vi "Set Cluster Element Disabled.vi"(6 "Disabled":T1(ring), 8 "error in":errorcluster, 9 "Class To Set":string, 10 "Index":i32, 11 "Cluster":refnum<vi>) -> (0 "error out":errorcluster, 3 "Cluster (dup)":refnum<vi>)   [LabVIEW 2015, in "Utility.lvlib"]
doc: "Used to set the Disabled property of an element of a cluster, referenced via the <b>Index</b> input.\n\nA special mode of operation of this VI is when <b>Index</b> is set to -1. In this case the disabled state is applied to all the controls in the cluster of the specific Class referenced by <b>Class To Set</b>. If this input is empty the class is ignored and the disabled state is applied to all the controls in the cluster. The <b>Class To Set</b> input is not case sensitive."
uses:
  Utility.lvlib
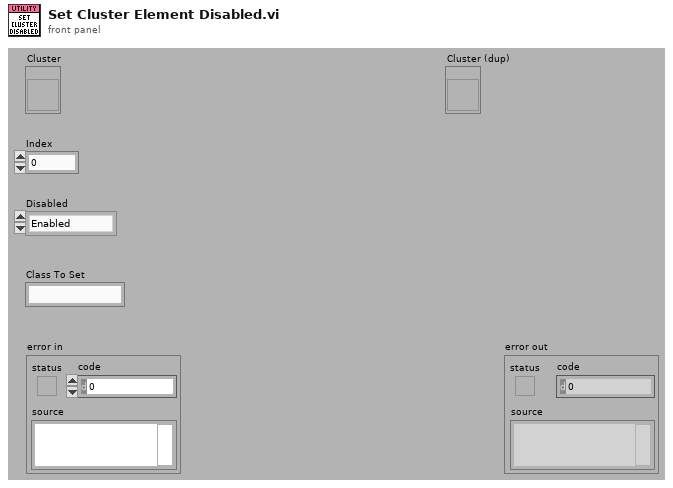
[diagram p1: front panel]
types:
  T1 = enum8{"Enabled", "Disabled", "Disabled and Grayed Out"}
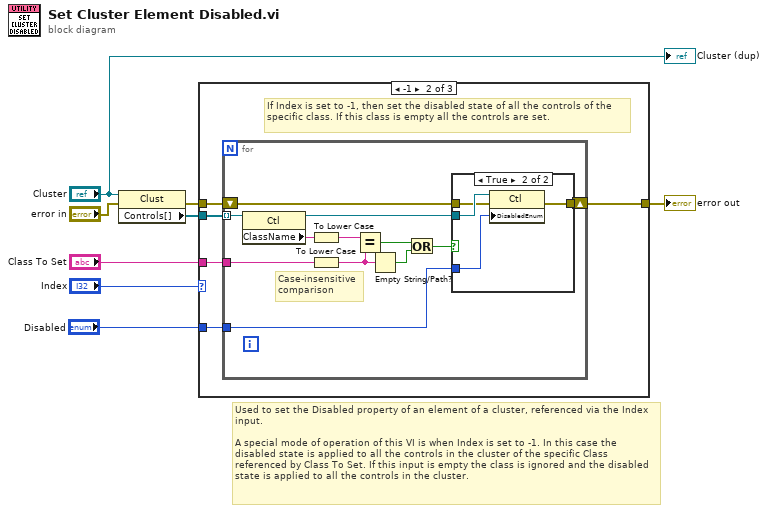
[diagram p0: block diagram]
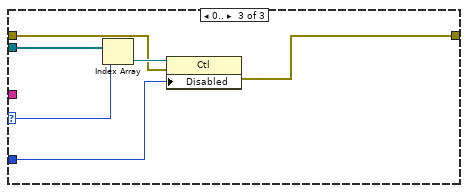
[diagram p4: hidden frame]
diagram:
  # "Used to set the Disabled property of an element of a cluster, referenced via the Index input.\n\nA special mode of operation of this VI is when Index is set to -1. In this case the disabled state is applied to all the controls in the cluster of the specific Class referenced by Class To Set. If this input is empty the class is ignored and the disabled state is applied to all the controls in the cluster."
  n1 = property class="Clust"(reference="Cluster", error in="error in") -> (error out=w6:errorcluster, "Controls[]"=w8:refnum<vi>[])  [unwired: 1 out]
  n2 = case shown="-1" "Index" {
    selector: "Index" -> [_ _ w32]
    tunnel: w8 -> [_ w14 w37]
    tunnel: "Disabled" -> [_ w13 w35]
    tunnel: w6 -> [w9 w12 w34]
    tunnel: [w9 w11 w33] -> w5
    tunnel: "Class To Set" -> [_ w10 _]
    frame Default {
      # "Bad input value for index. Do nothing"
    }
    frame -1 {
      # "If Index is set to -1, then set the disabled state of all the controls of the specific class. If this class is empty all the controls are set."
      n3 = for {
        tunnel: w14 -> [w25] mode=indexing
        tunnel: w13 -> [w15]
        shift-right: [w26] -> w11
        shift-left: w12 -> [w23]
        tunnel: w10 -> [w17]
        # "Case-insensitive comparison"
        n4 = property class="Ctl"(reference=w25) -> (reference out=w24:refnum<vi>, "ClassName"=w19:string)  [unwired: 1 in, 1 out]
        n5 = To Lower Case(string=w19) -> (all lower case string=w18:string)
        n6 = To Lower Case(string=w17) -> (all lower case string=w16:string)
        n7 = Equal?(x=w18, y=w16) -> (x = y?=w22:bool)
        n8 = Empty String/Path?(string/path=w16) -> (empty?=w21:bool)
        n9 = Or(x=w22, y=w21) -> (x .or. y?=w20:bool)
        n10 = case shown="True" w20 {
          tunnel: [w27 w31] -> w26
          tunnel: w24 -> [_ w30]
          tunnel: w23 -> [w27 w29]
          tunnel: w15 -> [_ w28]
          frame False {
          }
          frame True {
            n11 = property class="Ctl"(reference=w30, error in=w29, "DisabledEnum"=w28) -> (error out=w31:errorcluster)  [unwired: 1 out]
          }
        }
      }
    }
    frame 0.. {
      n12 = Index Array(array=w37, index=w32) -> (element=w36:refnum<vi>)
      n13 = property class="Ctl"(reference=w36, error in=w34, "Disabled"=w35) -> (error out=w33:errorcluster)  [unwired: 1 out]
    }
  }
  "error out" <- w5
  "Cluster (dup)" <- "Cluster"
